vi "Main_PIV_Alex.vi"() -> ()   [LabVIEW 2011]
uses:
  <vilib>/Utility/error.llb/DialogType.ctl
  <vilib>/DAQmx/write.llb/DAQmx Write (Digital Wfm 1Chan NSamp).vi
  <vilib>/DAQmx/write.llb/DAQmx Write (Digital Bool 1Line 1Point).vi
  <vilib>/Waveform/DWDTOps.llb/DWDT Boolean Array to Digital.vi
  <vilib>/DAQmx/create/channels.llb/DAQmx Create Channel (DO-Digital Output).vi
  <vilib>/DAQmx/configure/timing.llb/DAQmx Timing (Sample Clock).vi
  <vilib>/Waveform/DWDTOps.llb/DWDT Uncompress Digital.vi
  <vilib>/DAQmx/miscellaneous.llb/DAQmx Fill In Error Info.vi
  <vilib>/DAQmx/configure/trigger.llb/DAQmx Start Trigger (Digital Edge).vi
panel:
  in  "Tot # of fake flashes 2":i32=50
  out "Pulse Count 2":dbl=50.0
  in  "Loop Time (ms)":u32=100
  in  "Lines 3":tag="Dev1/port0/line0:7" caption="Lines"
  in  "I.C. rate  2":dbl=1000000.0 format="%0.2f"
  out "output array 3":bool[][](array[boolean])
  in  "Pulse 1 Delay 2":u32=500
  in  "On Time 1":u32=1000
  in  "Pulse 2 Delay 2":u32=1500
  in  "On Time 2":u32=1000
  in  "TSI Delay":u32=2
  in  "TSI On Time":u32=10
  out "Image Count":dbl=9.0
  in  "# of I.C. Images":i32=10
  in  "On Tim":u32=300
  in  "Laser 2 delay":u32=1960
  in  "On Time":u32=300
  in  "Laser 1 delay":u32=1910
  out "output array 4":bool[][](array[boolean])
  in  "I.C. Laser rate":dbl=1000000.0 format="%0.2f"
  in  "Lines 4":tag="Dev1/port0/line0:7" caption="Lines"
  in  "TSI":bool=TRUE
  in  "TSI Delay":u32=2
  in  "TSI On Time":u32=10
  in  "Ekspla Laser 2":bool=TRUE
  in  "Laser 2 Delay":u32=1960
  in  "Laser 2 On Time":u32=300
  in  "Ekspla Laser 1":bool=TRUE
  in  "Laser 1 Delay":u32=1910
  in  "Laser 1 On Time":u32=300
  in  "Tot # of fake flashes":i32=49
  out "Pulse Count":dbl=49.0
  in  "Lines 2":tag="Dev1/port0/line0:7" caption="Lines"
  in  "I.C. rate":dbl=1000000.0 format="%0.2f"
  out "output array 2":bool[][](array[boolean])
  in  "Loop Time (ms)":u32=100
  in  "Pulse 1 Delay":u32=500
  in  "On Time":u32=1000
  in  "Pulse 2 Delay":u32=1500
  in  "On Time":u32=1000
  in  "Laser 2 (Fire)":bool
  in  "Laser 1 (Fire)":bool
  in  "FAVs":bool
  in  "Test Trigger":bool
  in  "QS1 On Time":u32
  in  "QS1 Delay":u32
  in  "Fire2 On Time":u32
  in  "Fire2 Delay 3":u32
  in  "QS2 On Time":u32
  in  "QS2 Delay":u32
  in  "Fire1 On Time":u32
  in  "Fire1 Delay 3":u32
  out "output array":bool[][](array[boolean])
  out "Digital Waveform (PCI 6534)":digitalwaveform(graph)={"t0"=timestamp(0 s since 1904-01-01), "dt"=1e-06, "Y"={"transitions"=[], "data"=array3000x8[24000 elements]}}
  in  "Fire Rate":dbl=1000000.0 format="%0.2f"
  in  "Lines":tag="Dev1/port0/line0:7"
  in  "Boolean 24":bool
  in  "End Wall Valve":bool
  in  "Lower Tube E4":bool
  in  "DING":bool
  in  "Lower Tueb E2":bool
  in  "Lowr Tube E1":bool
  in  "Boolean 18":bool
  in  "Boolean 17":bool
  in  "Boolean 16":bool
  in  "Tube LP TV":bool
  in  "Fav #2":bool
  in  "Fav #1":bool
  in  "Vacuum Pump":bool
  in  "Boolean 11":bool
  in  "Diaph Vacuum":bool
  in  "Diaph Supply":bool
  in  "Diaph Vent":bool
  in  "Diaph Master":bool
  in  "Driver LP TV":bool
  in  "Supply Auto V":bool
  in  "Driver Vacuum":bool
  in  "Driver Supply":bool
  in  "Driver Vent":bool
  in  "Driver Master":bool
  in  "stop":bool
  in  "Run Experiment":bool
  # "Shock Tube Controls"
  # "Injectors"
  # "BubbleFill"
  # "Initial Conditions"
  # "Experiment"
  # "SureliteII (need a charge pulse)"
  # "Qswitch/Fire delay: 194us"
  # "Ekspla Charge I.C. (49 fake pulses)"
  # "Fire ---> Qswitch"
  # "i.e. 49"
  # "SureliteII (not needed)"
  # "IC Images"
  # "Ekspla Fire"
  # "TSI"
  # "lase at: 3264 and 3314"
  # "readout time before shock"
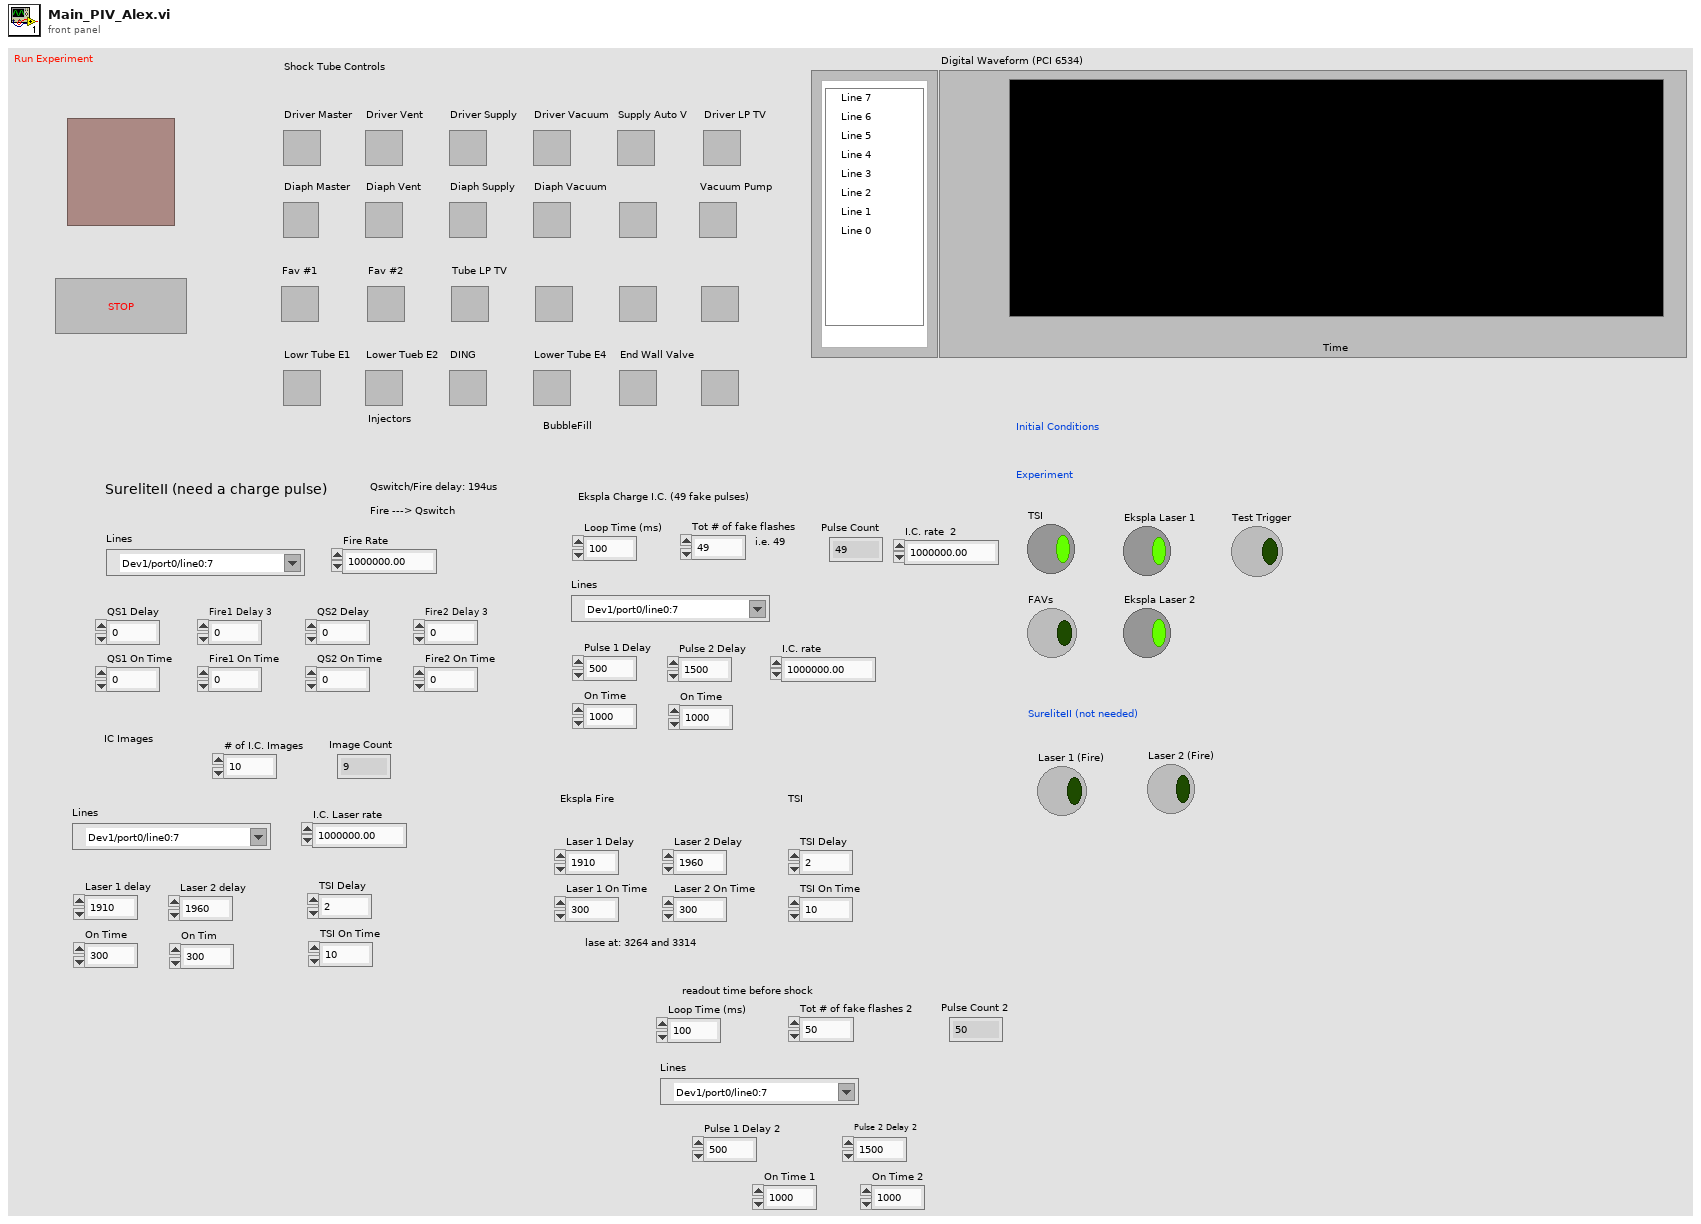
[diagram p1: front panel]
types:
  T1 = typedef "DialogType.ctl" = u16
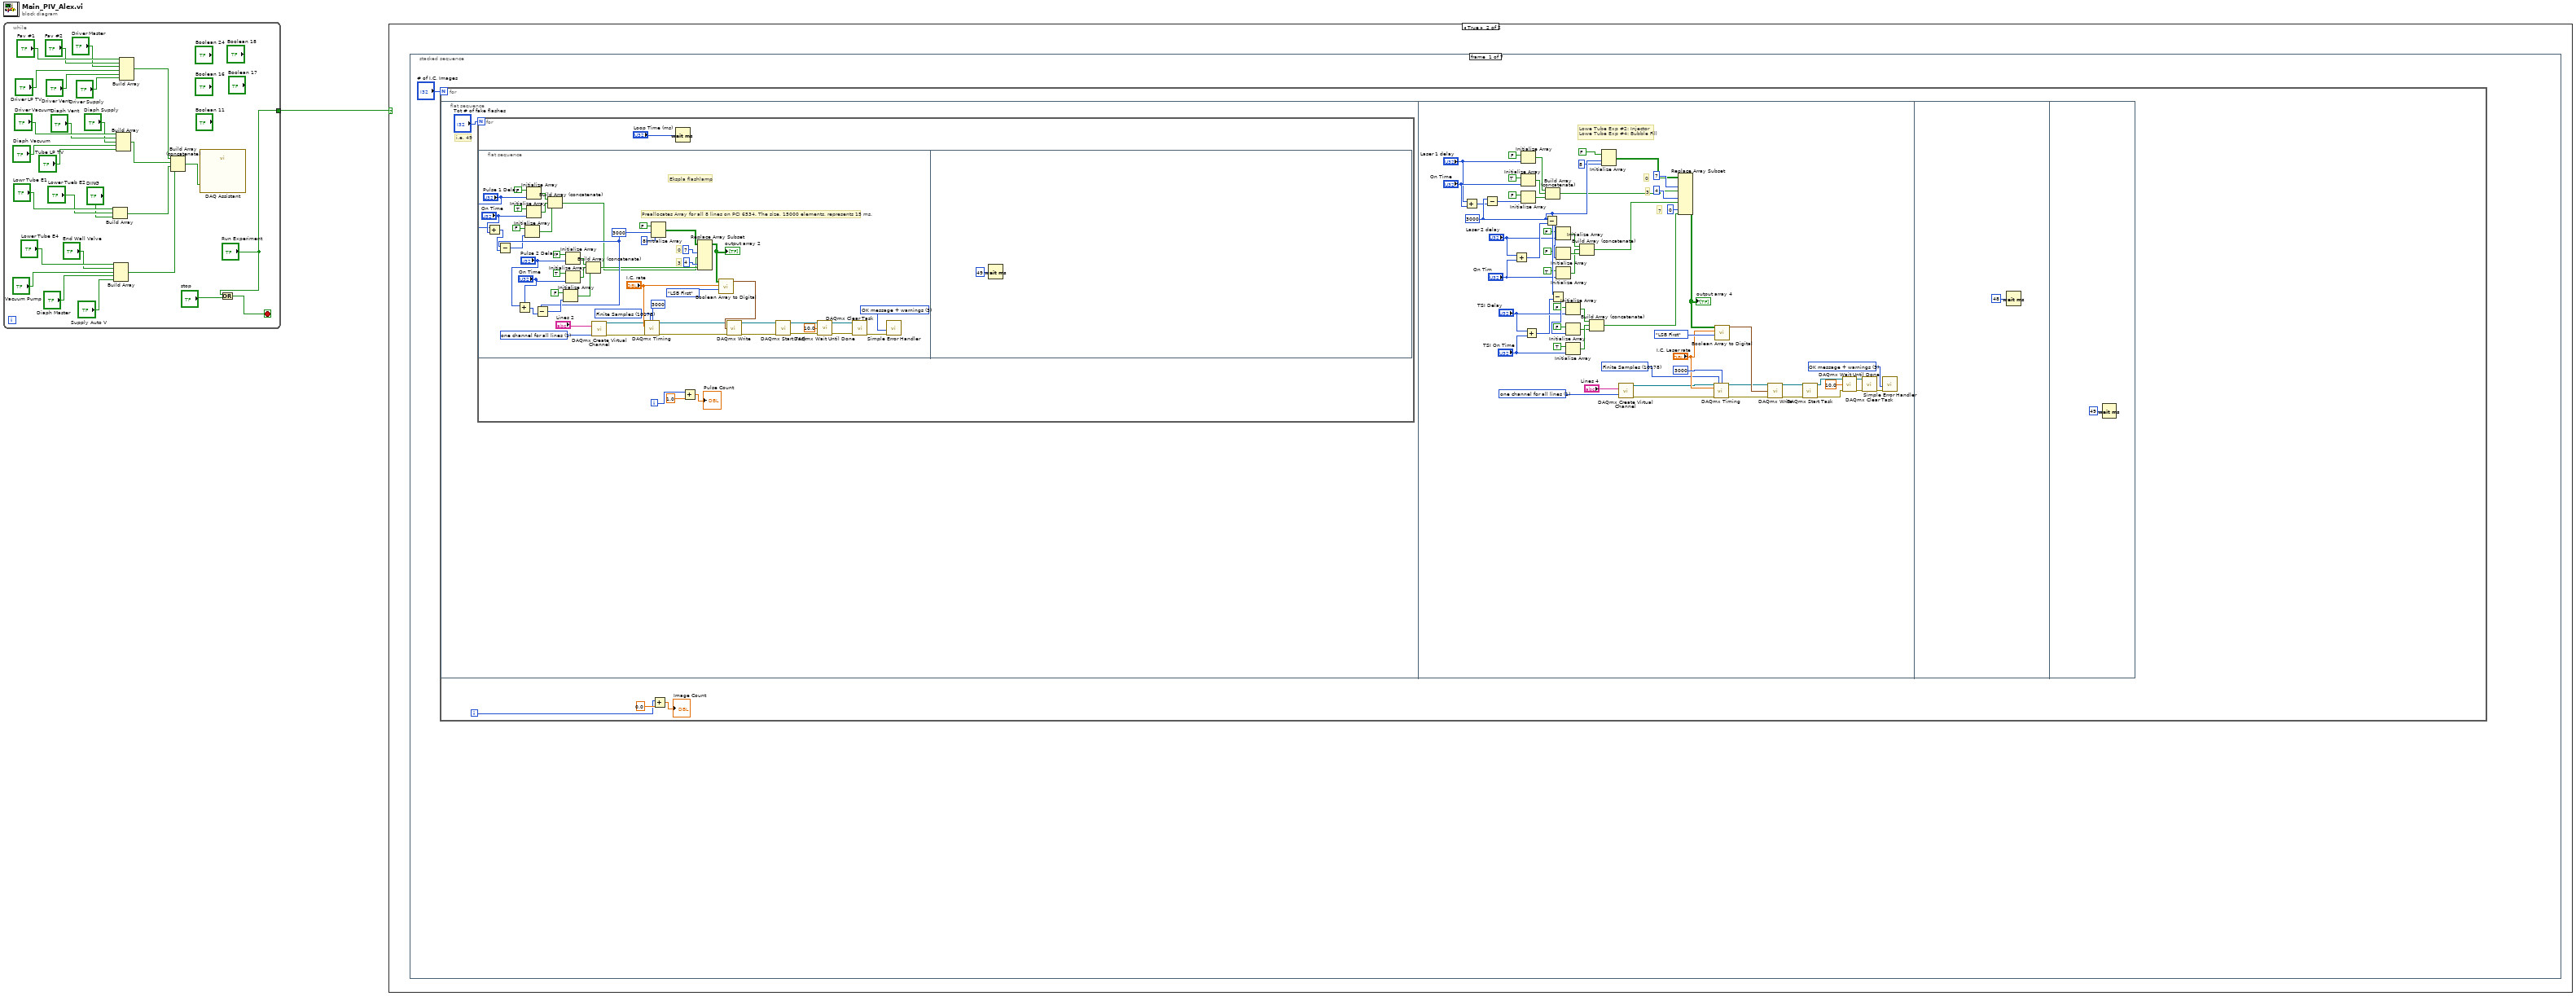
[diagram p0: block diagram]
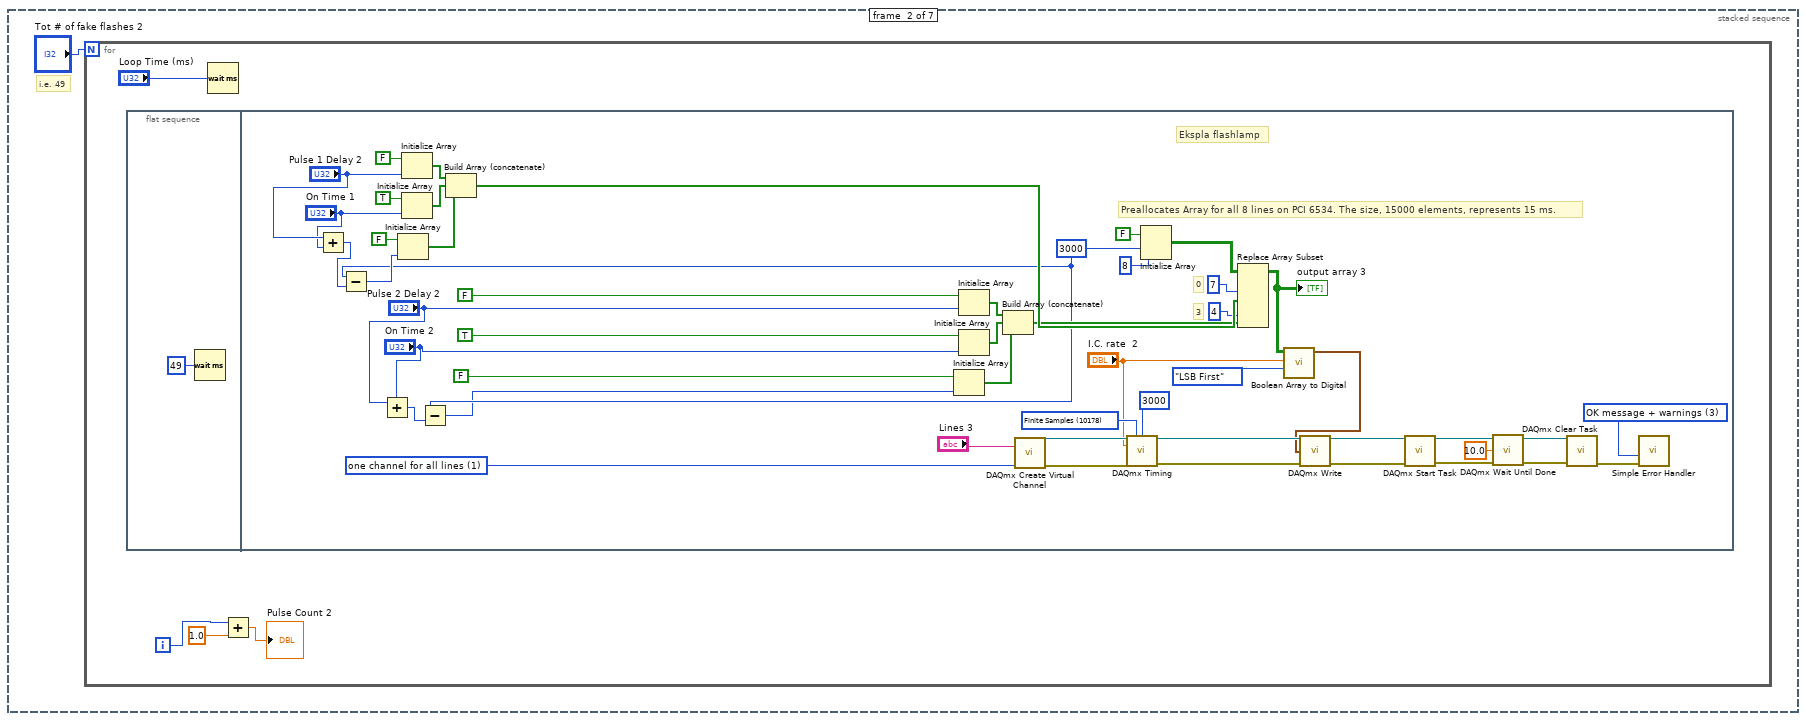
[diagram p3: hidden frame]
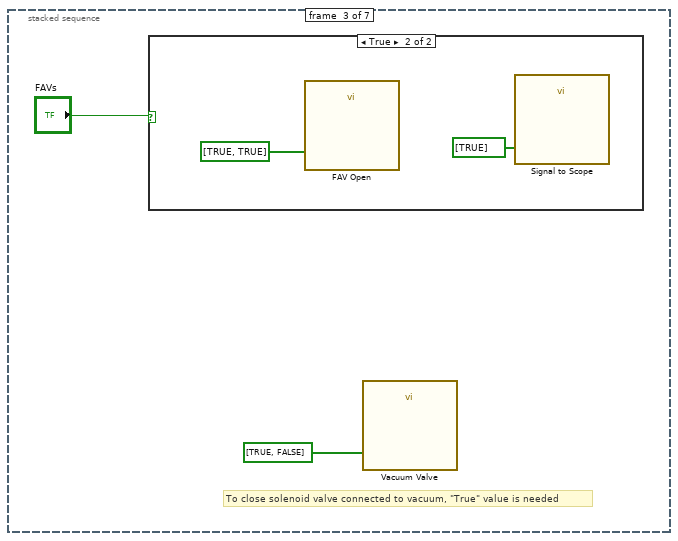
[diagram p4: hidden frame]
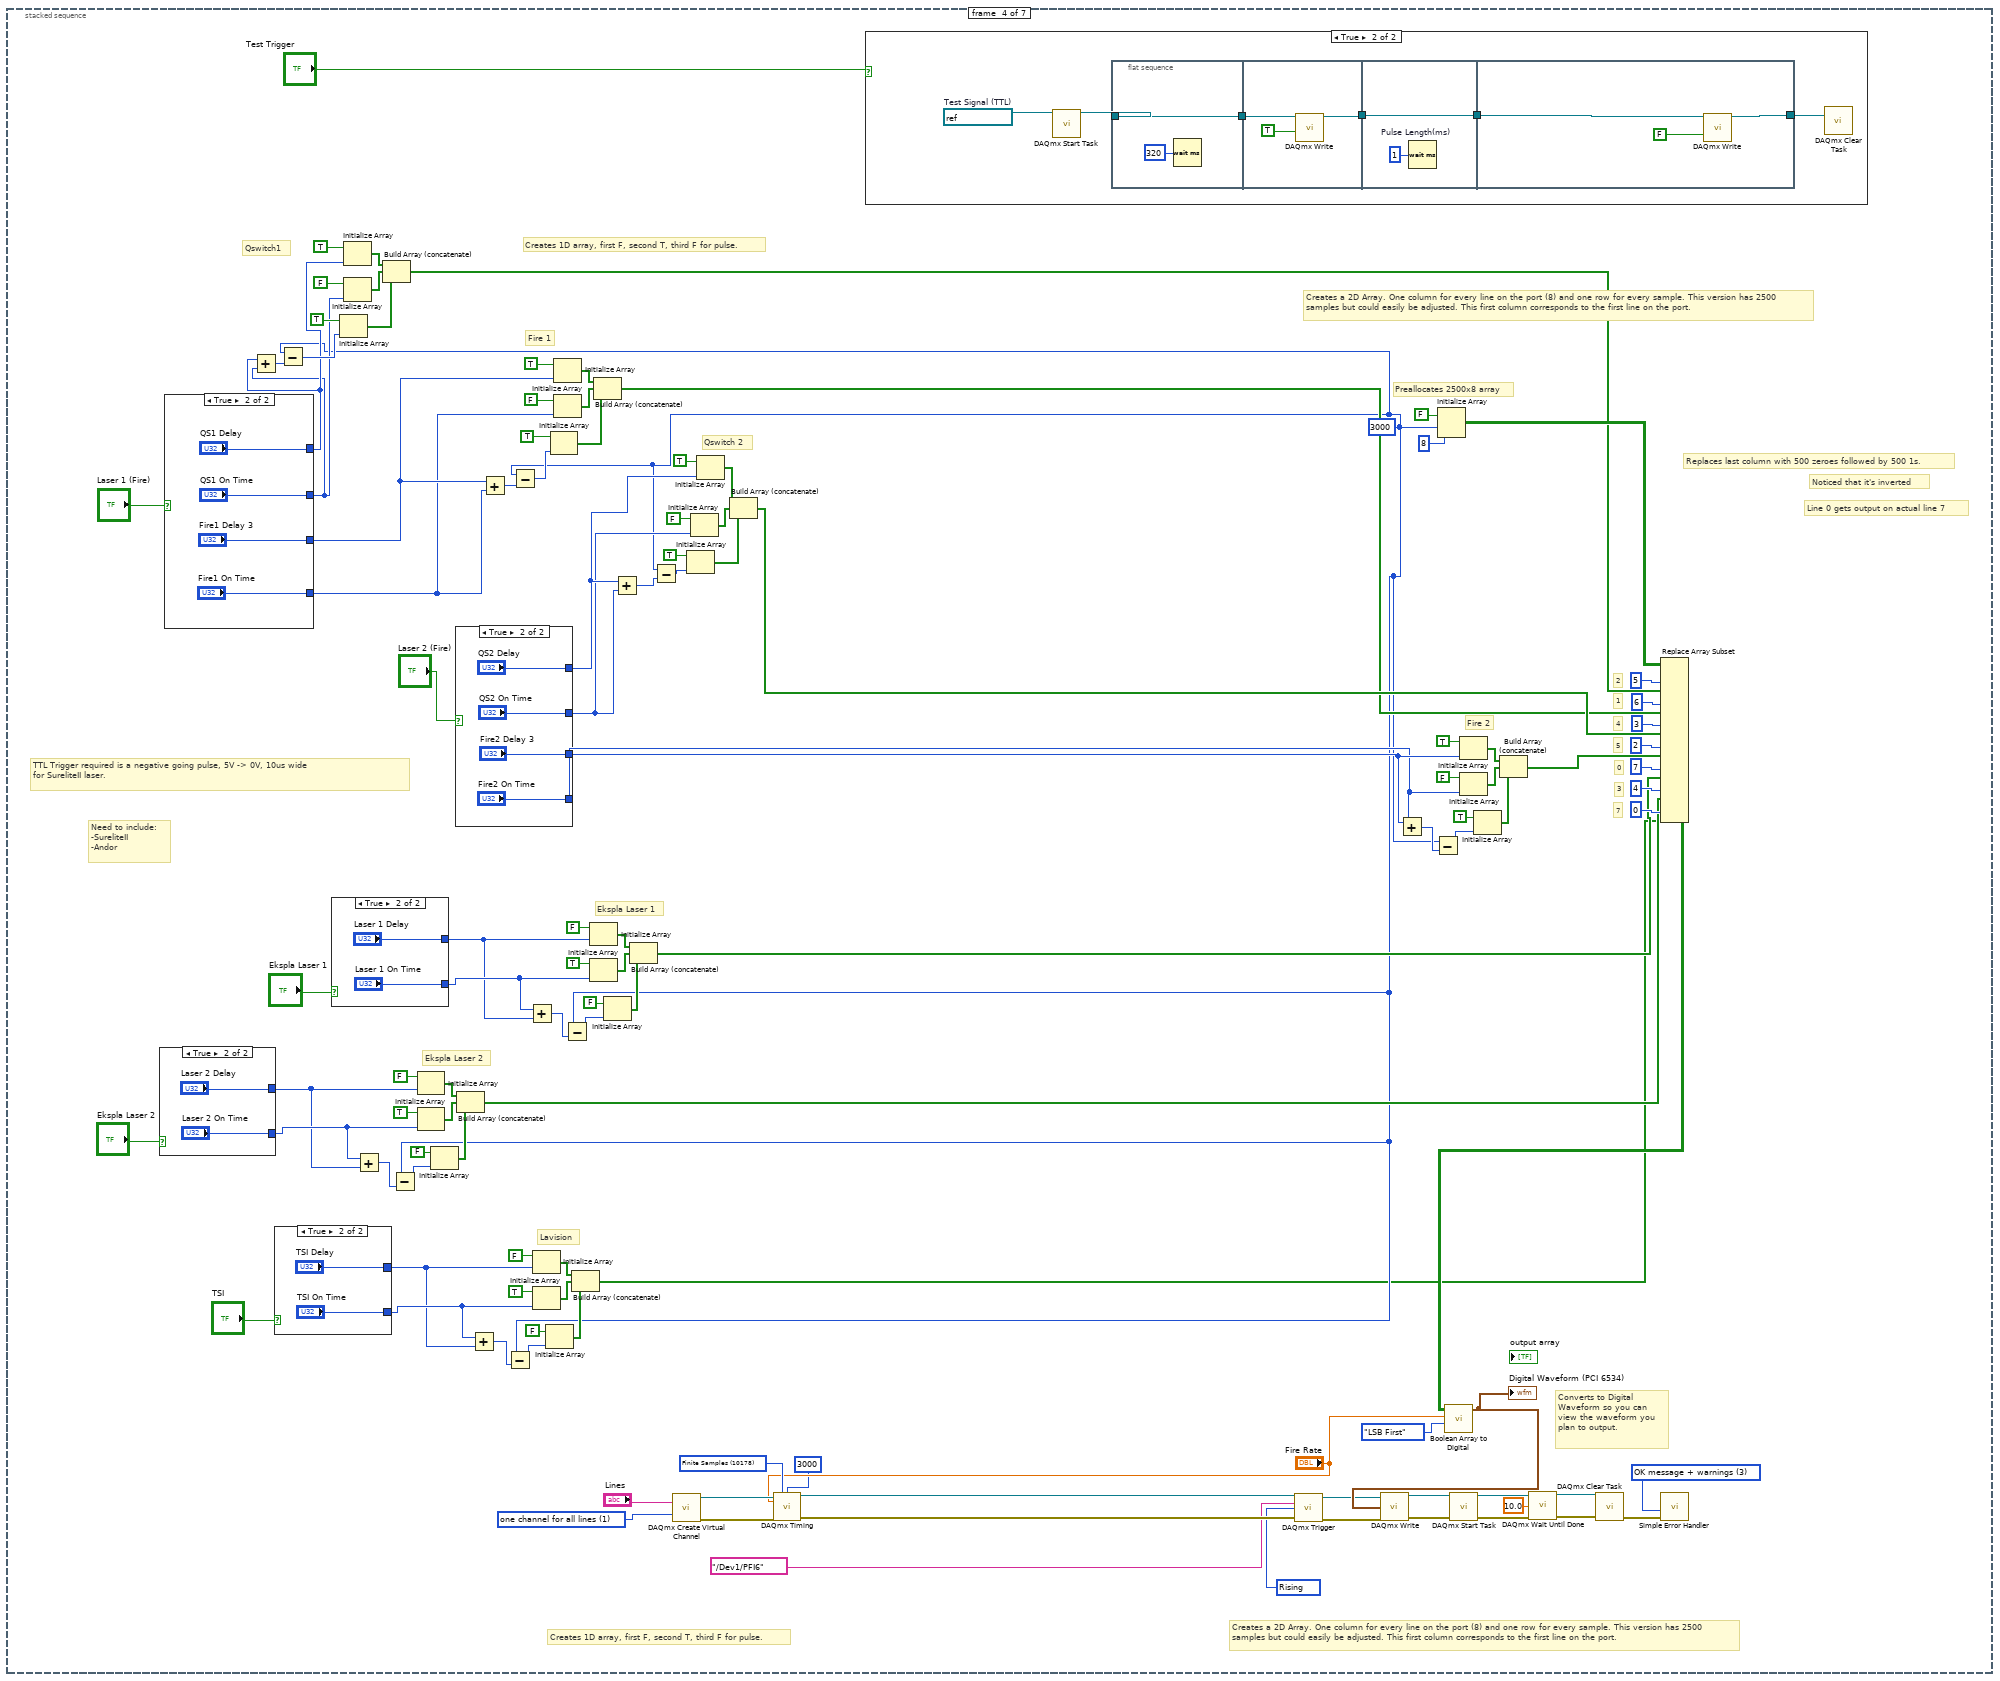
[diagram p6: hidden frame]
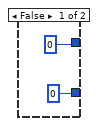
[diagram p7: hidden frame]
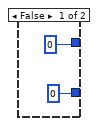
[diagram p8: hidden frame]
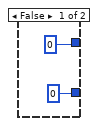
[diagram p9: hidden frame]
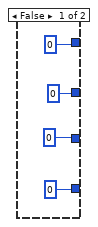
[diagram p10: hidden frame]
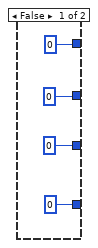
[diagram p11: hidden frame]
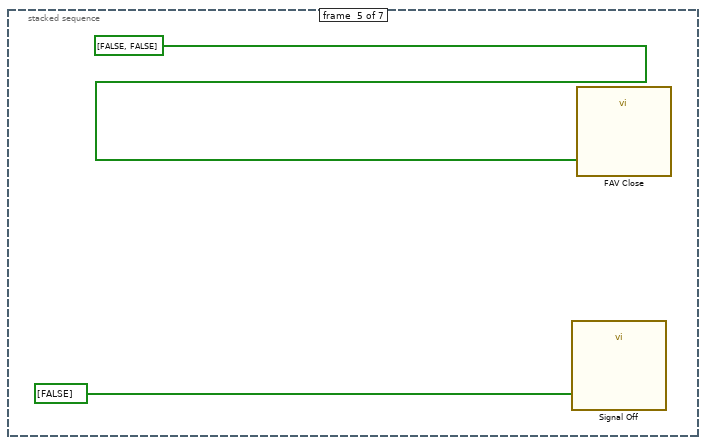
[diagram p13: hidden frame]
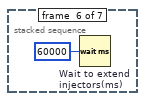
[diagram p14: hidden frame]
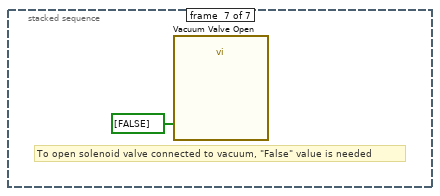
[diagram p15: hidden frame]
diagram:
  n1 = while {
    tunnel: ["Run Experiment"] -> w1
    stop <- w26 stop-if-true
    n2 = Build Array("Lowr Tube E1", "Lower Tueb E2", "DING") -> (w23:bool[])
    n3 = Build Array("Lower Tube E4", "End Wall Valve", "Vacuum Pump", "Diaph Master", "Supply Auto V") -> (w22:bool[])
    n4 = Build Array("Driver Vacuum", "Diaph Vent", "Diaph Supply", "Diaph Vacuum", "Tube LP TV") -> (w24:bool[])
    n5 = Build Array("Fav #1", "Fav #2", "Driver Master", "Driver LP TV", "Driver Vent", "Driver Supply") -> (w25:bool[])
    n6 = Build Array (concatenate)(w25, w24, w23, w22) -> (w2:bool[])
    n7 = call "DAQ Assistant"("data"=w2) -> ()  [unwired: 17 in, 2 out]
    n8 = Or(x="Run Experiment", y="stop") -> (x .or. y?=w26:bool)
  }
  n9 = case shown="True" w1 {
    frame False {
    }
    frame True {
      n10 = stacked-sequence {
        frame #0 {
          n11 = for {
            N: "# of I.C. Images" -> [_]
            i -> [w30]
            n12 = flat-sequence {
              frame #0 {
                # "i.e. 49"
                n13 = for {
                  N: "Tot # of fake flashes" -> [_]
                  i -> [w36]
                  n14 = flat-sequence {
                    frame #0 {
                      w85 = 3000 ("dimension size")
                      w44 = 10178 items=["Finite Samples"=10178, "Continuous Samples"=10123, "Hardware Timed Single Point"=12522] ("sample mode")
                      w41 = 1 items=["one channel for each line", "one channel for all lines"] ("line grouping")
                      w40 = T1 3 items=["no dialog", "OK message", "continue or stop message", "OK message + warnings", "continue/stop + warnings"] ("type of dialog (OK msg:1)")
                      # "0"
                      # "3"
                      # "Ekspla flashlamp"
                      # "Preallocates Array for all 8 lines on PCI 6534. The size, 15000 elements, represents 15 ms."
                      n15 = Add(x="Pulse 1 Delay", y="On Time") -> (x+y=w80:u32)
                      n16 = Subtract(x=w85, y=w80) -> (x-y=w81:u32)
                      n17 = Add(x="Pulse 2 Delay", y="On Time") -> (x+y=w84:u32)
                      n18 = Initialize Array(FALSE, w81) -> (w69:bool[])
                      n19 = Initialize Array(FALSE, "Pulse 1 Delay") -> (w58:bool[])
                      n20 = Initialize Array(TRUE, "On Time") -> (w57:bool[])
                      n21 = Subtract(x=w85, y=w84) -> (x-y=w86:u32)
                      n22 = Build Array (concatenate)(w58, w57, w69) -> (w59:bool[])
                      n23 = Initialize Array(FALSE, w86) -> (w75:bool[])
                      n24 = Initialize Array(FALSE, "Pulse 2 Delay") -> (w73:bool[])
                      n25 = Initialize Array(TRUE, "On Time") -> (w72:bool[])
                      n26 = Build Array (concatenate)(w73, w72, w75) -> (w77:bool[])
                      n27 = call-poly <vilib>:"DAQmx Create Virtual Channel.vi"("lines"="Lines 2", "line grouping"=w41) -> ("task out"=w42:refnum<k21>, "error out"=w43:errorcluster)  [unwired: 12 in]
                      n28 = call-poly <vilib>:"DAQmx Timing.vi"("task/channels in"=w42, "sample mode"=w44, "samples per channel"=3000, "rate"="I.C. rate", "error in"=w43) -> ("task out"=w54:refnum<k21>, "error out"=w55:errorcluster)  [unwired: 9 in]
                      n29 = Initialize Array(FALSE, w85, 8 ("dimension size")) -> (w48:bool[][])
                      n30 = Replace Array Subset(array=w48, new element #1=w59, index (col) #1=7 ("disabled index (col)"), new element #2=w77, index (col) #2=4 ("index (col)")) -> (w51:bool[][])  [unwired: 2 in]
                      "output array 2" <- w51
                      n31 = call-poly <vilib>:"Boolean Array to Digital.vi"("mode"=enum16{"LSB First", "MSB First"}."LSB First", "sample rate"="I.C. rate", "boolean array"=w51) -> ("digital waveform"=w61:digitalwaveform)  [unwired: 7 in, 1 out]
                      n32 = call-poly <vilib>:"DAQmx Write.vi"("task/channels in"=w54, "data"=w61, "error in"=w55) -> ("task out"=w52:refnum<k21>, "error out"=w53:errorcluster)  [unwired: 10 in, 1 out]
                      n33 = call <vilib>:"DAQmx Start Task.vi"("task/channels in"=w52, "error in"=w53) -> ("task out"=w65:refnum<k21>, "error out"=w66:errorcluster)  [unwired: 12 in]
                      n34 = call <vilib>:"DAQmx Wait Until Done.vi"("task/channels in"=w65, "timeout (sec)"=10.0, "error in"=w66) -> ("task out"=w63:refnum<k21>, "error out"=w62:errorcluster)  [unwired: 11 in]
                      n35 = call <vilib>:"DAQmx Clear Task.vi"("task in"=w63, "error in"=w62) -> ("error out"=w38:errorcluster)  [unwired: 13 in]
                      n36 = call <vilib>:"Simple Error Handler.vi"("type of dialog (OK msg:1)"=w40, "error in (no error)"=w38) -> ()  [unwired: 3 in, 5 out]
                    }
                    frame #1 {
                      n37 = Wait (ms)(milliseconds to wait=u32 49) -> ()  [unwired: 1 out]
                    }
                  }
                  n38 = Wait (ms)(milliseconds to wait="Loop Time (ms)") -> ()  [unwired: 1 out]
                  n39 = Add(x=w36, y=1.0) -> (x+y=→"Pulse Count":dbl)
                }
              }
              frame #1 {
                w146 = 3000 ("dimension size")
                w94 = 10178 items=["Finite Samples"=10178, "Continuous Samples"=10123, "Hardware Timed Single Point"=12522] ("sample mode")
                w91 = 1 items=["one channel for each line", "one channel for all lines"] ("line grouping")
                w90 = T1 3 items=["no dialog", "OK message", "continue or stop message", "OK message + warnings", "continue/stop + warnings"] ("type of dialog (OK msg:1)")
                # "7"
                # "0"
                # "3"
                # "Lowe Tube Exp #2: Injector\nLowe Tube Exp #4: Bubble Fill"
                n40 = Add(x="Laser 1 delay", y="On Time") -> (x+y=w130:u32)
                n41 = Subtract(x=w146, y=w130) -> (x-y=w131:u32)
                n42 = Add(x="Laser 2 delay", y="On Tim") -> (x+y=w134:u32)
                n43 = Initialize Array(FALSE, "Laser 1 delay") -> (w108:bool[])
                n44 = Initialize Array(TRUE, "On Time") -> (w107:bool[])
                n45 = Initialize Array(FALSE, w131) -> (w119:bool[])
                n46 = Add(x="TSI Delay", y="TSI On Time") -> (x+y=w135:u32)
                n47 = Subtract(x=w146, y=w134) -> (x-y=w144:u32)
                n48 = Build Array (concatenate)(w108, w107, w119) -> (w109:bool[])
                n49 = Subtract(x=w146, y=w135) -> (x-y=w145:u32)
                n50 = Initialize Array(FALSE, "Laser 2 delay") -> (w123:bool[])
                n51 = Initialize Array(FALSE, w144) -> (w125:bool[])
                n52 = Initialize Array(TRUE, "On Tim") -> (w122:bool[])
                n53 = Initialize Array(FALSE, "TSI Delay") -> (w140:bool[])
                n54 = Initialize Array(FALSE, w145) -> (w138:bool[])
                n55 = Initialize Array(TRUE, "TSI On Time") -> (w141:bool[])
                n56 = Build Array (concatenate)(w123, w122, w125) -> (w127:bool[])
                n57 = Build Array (concatenate)(w140, w141, w138) -> (w147:bool[])
                n58 = Initialize Array(FALSE, w146, 8 ("dimension size")) -> (w98:bool[][])
                n59 = call-poly <vilib>:"DAQmx Create Virtual Channel.vi"("lines"="Lines 4", "line grouping"=w91) -> ("task out"=w92:refnum<k21>, "error out"=w93:errorcluster)  [unwired: 12 in]
                n60 = Replace Array Subset(array=w98, new element #1=w109, index (col) #1=7 ("disabled index (col)"), new element #2=w127, index (col) #2=4 ("index (col)"), new element #3=w147, index (col) #3=0 ("index (col)")) -> (w101:bool[][])  [unwired: 3 in]
                "output array 4" <- w101
                n61 = call-poly <vilib>:"DAQmx Timing.vi"("task/channels in"=w92, "sample mode"=w94, "samples per channel"=3000, "rate"="I.C. Laser rate", "error in"=w93) -> ("task out"=w104:refnum<k21>, "error out"=w105:errorcluster)  [unwired: 9 in]
                n62 = call-poly <vilib>:"Boolean Array to Digital.vi"("mode"=enum16{"LSB First", "MSB First"}."LSB First", "sample rate"="I.C. Laser rate", "boolean array"=w101) -> ("digital waveform"=w111:digitalwaveform)  [unwired: 7 in, 1 out]
                n63 = call-poly <vilib>:"DAQmx Write.vi"("task/channels in"=w104, "data"=w111, "error in"=w105) -> ("task out"=w102:refnum<k21>, "error out"=w103:errorcluster)  [unwired: 10 in, 1 out]
                n64 = call <vilib>:"DAQmx Start Task.vi"("task/channels in"=w102, "error in"=w103) -> ("task out"=w115:refnum<k21>, "error out"=w116:errorcluster)  [unwired: 12 in]
                n65 = call <vilib>:"DAQmx Wait Until Done.vi"("task/channels in"=w115, "timeout (sec)"=10.0, "error in"=w116) -> ("task out"=w113:refnum<k21>, "error out"=w112:errorcluster)  [unwired: 11 in]
                n66 = call <vilib>:"DAQmx Clear Task.vi"("task in"=w113, "error in"=w112) -> ("error out"=w88:errorcluster)  [unwired: 13 in]
                n67 = call <vilib>:"Simple Error Handler.vi"("type of dialog (OK msg:1)"=w90, "error in (no error)"=w88) -> ()  [unwired: 3 in, 5 out]
              }
              frame #2 {
                n68 = Wait (ms)(milliseconds to wait=u32 48) -> ()  [unwired: 1 out]
              }
              frame #3 {
                n69 = Wait (ms)(milliseconds to wait=u32 49) -> ()  [unwired: 1 out]
              }
            }
            n70 = Add(x=w30, y=0.0) -> (x+y=→"Image Count":dbl)
          }
        }
        frame #1 {
          # "i.e. 49"
          n71 = for {
            N: "Tot # of fake flashes 2" -> [_]
            i -> [w154]
            n72 = flat-sequence {
              frame #0 {
                n73 = Wait (ms)(milliseconds to wait=u32 49) -> ()  [unwired: 1 out]
              }
              frame #1 {
                w158 = 3000 ("dimension size")
                w199 = 10178 items=["Finite Samples"=10178, "Continuous Samples"=10123, "Hardware Timed Single Point"=12522] ("sample mode")
                w202 = 1 items=["one channel for each line", "one channel for all lines"] ("line grouping")
                w203 = T1 3 items=["no dialog", "OK message", "continue or stop message", "OK message + warnings", "continue/stop + warnings"] ("type of dialog (OK msg:1)")
                # "0"
                # "3"
                # "Ekspla flashlamp"
                # "Preallocates Array for all 8 lines on PCI 6534. The size, 15000 elements, represents 15 ms."
                n74 = Add(x="Pulse 1 Delay 2", y="On Time 1") -> (x+y=w163:u32)
                n75 = Subtract(x=w158, y=w163) -> (x-y=w162:u32)
                n76 = Add(x="Pulse 2 Delay 2", y="On Time 2") -> (x+y=w159:u32)
                n77 = Initialize Array(FALSE, w162) -> (w174:bool[])
                n78 = Initialize Array(FALSE, "Pulse 1 Delay 2") -> (w185:bool[])
                n79 = Initialize Array(TRUE, "On Time 1") -> (w186:bool[])
                n80 = Subtract(x=w158, y=w159) -> (x-y=w157:u32)
                n81 = Build Array (concatenate)(w185, w186, w174) -> (w184:bool[])
                n82 = Initialize Array(FALSE, w157) -> (w168:bool[])
                n83 = Initialize Array(FALSE, "Pulse 2 Delay 2") -> (w170:bool[])
                n84 = Initialize Array(TRUE, "On Time 2") -> (w171:bool[])
                n85 = Build Array (concatenate)(w170, w171, w168) -> (w166:bool[])
                n86 = call-poly <vilib>:"DAQmx Create Virtual Channel.vi"("lines"="Lines 3", "line grouping"=w202) -> ("task out"=w201:refnum<k21>, "error out"=w200:errorcluster)  [unwired: 12 in]
                n87 = call-poly <vilib>:"DAQmx Timing.vi"("task/channels in"=w201, "sample mode"=w199, "samples per channel"=3000, "rate"="I.C. rate  2", "error in"=w200) -> ("task out"=w189:refnum<k21>, "error out"=w188:errorcluster)  [unwired: 9 in]
                n88 = Initialize Array(FALSE, w158, 8 ("dimension size")) -> (w195:bool[][])
                n89 = Replace Array Subset(array=w195, new element #1=w184, index (col) #1=7 ("disabled index (col)"), new element #2=w166, index (col) #2=4 ("index (col)")) -> (w192:bool[][])  [unwired: 2 in]
                "output array 3" <- w192
                n90 = call-poly <vilib>:"Boolean Array to Digital.vi"("mode"=enum16{"LSB First", "MSB First"}."LSB First", "sample rate"="I.C. rate  2", "boolean array"=w192) -> ("digital waveform"=w182:digitalwaveform)  [unwired: 7 in, 1 out]
                n91 = call-poly <vilib>:"DAQmx Write.vi"("task/channels in"=w189, "data"=w182, "error in"=w188) -> ("task out"=w191:refnum<k21>, "error out"=w190:errorcluster)  [unwired: 10 in, 1 out]
                n92 = call <vilib>:"DAQmx Start Task.vi"("task/channels in"=w191, "error in"=w190) -> ("task out"=w178:refnum<k21>, "error out"=w177:errorcluster)  [unwired: 12 in]
                n93 = call <vilib>:"DAQmx Wait Until Done.vi"("task/channels in"=w178, "timeout (sec)"=10.0, "error in"=w177) -> ("task out"=w180:refnum<k21>, "error out"=w181:errorcluster)  [unwired: 11 in]
                n94 = call <vilib>:"DAQmx Clear Task.vi"("task in"=w180, "error in"=w181) -> ("error out"=w205:errorcluster)  [unwired: 13 in]
                n95 = call <vilib>:"Simple Error Handler.vi"("type of dialog (OK msg:1)"=w203, "error in (no error)"=w205) -> ()  [unwired: 3 in, 5 out]
              }
            }
            n96 = Wait (ms)(milliseconds to wait="Loop Time (ms)") -> ()  [unwired: 1 out]
            n97 = Add(x=w154, y=1.0) -> (x+y=→"Pulse Count 2":dbl)
          }
        }
        frame #2 {
          # "To close solenoid valve connected to vacuum, \"True\" value is needed"
          n98 = case shown="True" "FAVs" {
            frame False {
            }
            frame True {
              n99 = call "FAV Open"("data"=bool[] [TRUE, TRUE]) -> ()  [unwired: 17 in, 2 out]
              n100 = call "Signal to Scope"("data"=bool[] [TRUE]) -> ()  [unwired: 17 in, 2 out]
            }
          }
          n101 = call "Vacuum Valve"("data"=bool[] [TRUE, FALSE]) -> ()  [unwired: 17 in, 2 out]
        }
        frame #3 {
          w281 = 10280 items=["Rising"=10280, "Falling"=10171] ("slope")
          w211 = 3000 ("dimension size")
          w322 = 10178 items=["Finite Samples"=10178, "Continuous Samples"=10123, "Hardware Timed Single Point"=12522] ("sample mode")
          w325 = 1 items=["one channel for each line", "one channel for all lines"] ("line grouping")
          w326 = T1 3 items=["no dialog", "OK message", "continue or stop message", "OK message + warnings", "continue/stop + warnings"] ("type of dialog (OK msg:1)")
          # "Lavision"
          # "Ekspla Laser 2"
          # "Ekspla Laser 1"
          # "7"
          # "3"
          # "0"
          # "Creates 1D array, first F, second T, third F for pulse."
          # "Creates a 2D Array. One column for every line on the port (8) and one row for every sample. This version has 2500 samples but could easily be adjusted. This first column corresponds to the first line on the port."
          # "Need to include:\n-SureliteII\n-Andor"
          # "4"
          # "1"
          # "2"
          # "5"
          # "TTL Trigger required is a negative going pulse, 5V -> 0V, 10us wide\nfor SureliteII laser."
          # "Fire 2"
          # "Qswitch 2"
          # "Fire 1"
          # "Qswitch1"
          # "Line 0 gets output on actual line 7"
          # "Noticed that it's inverted"
          # "Converts to Digital Waveform so you can view the waveform you plan to output."
          # "Creates 1D array, first F, second T, third F for pulse."
          # "Replaces last column with 500 zeroes followed by 500 1s."
          # "Preallocates 2500x8 array"
          # "Creates a 2D Array. One column for every line on the port (8) and one row for every sample. This version has 2500 samples but could easily be adjusted. This first column corresponds to the first line on the port."
          n102 = case shown="True" "Ekspla Laser 2" {
            tunnel: [0 "Laser 2 Delay"] -> w224
            tunnel: [0 "Laser 2 On Time"] -> w225
            frame False {
            }
            frame True {
            }
          }
          n103 = case shown="True" "Laser 1 (Fire)" {
            tunnel: [0 "QS1 Delay"] -> w259
            tunnel: [0 "QS1 On Time"] -> w258
            tunnel: [0 "Fire1 Delay 3"] -> w257
            tunnel: [0 "Fire1 On Time"] -> w256
            frame False {
            }
            frame True {
            }
          }
          n104 = Add(x=w259, y=w258) -> (x+y=w263:u32)
          n105 = case shown="True" "TSI" {
            tunnel: [0 "TSI Delay"] -> w213
            tunnel: [0 "TSI On Time"] -> w214
            frame False {
            }
            frame True {
            }
          }
          n106 = Subtract(x=w211, y=w263) -> (x-y=w262:u32)
          n107 = case shown="True" "Ekspla Laser 1" {
            tunnel: [0 "Laser 1 Delay"] -> w236
            tunnel: [0 "Laser 1 On Time"] -> w237
            frame False {
            }
            frame True {
            }
          }
          n108 = Initialize Array(TRUE, w262) -> (w264:bool[])
          n109 = Initialize Array(TRUE, w259) -> (w266:bool[])
          n110 = Initialize Array(FALSE, w258) -> (w267:bool[])
          n111 = Add(x=w225, y=w224) -> (x+y=w228:u32)
          n112 = Build Array (concatenate)(w266, w267, w264) -> (w261:bool[])
          n113 = Subtract(x=w211, y=w228) -> (x-y=w227:u32)
          n114 = Initialize Array(FALSE, w224) -> (w231:bool[])
          n115 = Initialize Array(TRUE, w225) -> (w232:bool[])
          n116 = Initialize Array(FALSE, w227) -> (w229:bool[])
          n117 = case shown="True" "Laser 2 (Fire)" {
            tunnel: [0 "QS2 Delay"] -> w254
            tunnel: [0 "QS2 On Time"] -> w253
            tunnel: [0 "Fire2 Delay 3"] -> w252
            tunnel: [0 "Fire2 On Time"] -> w251
            frame False {
            }
            frame True {
            }
          }
          n118 = Build Array (concatenate)(w231, w232, w229) -> (w223:bool[])
          n119 = Add(x=w214, y=w213) -> (x+y=w212:u32)
          n120 = Add(x=w257, y=w256) -> (x+y=w286:u32)
          n121 = Subtract(x=w211, y=w212) -> (x-y=w216:u32)
          n122 = Subtract(x=w211, y=w286) -> (x-y=w285:u32)
          n123 = Add(x=w237, y=w236) -> (x+y=w240:u32)
          n124 = Initialize Array(FALSE, w213) -> (w219:bool[])
          n125 = Initialize Array(TRUE, w214) -> (w220:bool[])
          n126 = Initialize Array(FALSE, w216) -> (w217:bool[])
          n127 = Initialize Array(TRUE, w285) -> (w299:bool[])
          n128 = Initialize Array(TRUE, w257) -> (w301:bool[])
          n129 = Initialize Array(FALSE, w256) -> (w302:bool[])
          n130 = Subtract(x=w211, y=w240) -> (x-y=w239:u32)
          n131 = Build Array (concatenate)(w219, w220, w217) -> (w210:bool[])
          n132 = Initialize Array(FALSE, w236) -> (w243:bool[])
          n133 = Initialize Array(TRUE, w237) -> (w244:bool[])
          n134 = Build Array (concatenate)(w301, w302, w299) -> (w282:bool[])
          n135 = Initialize Array(FALSE, w239) -> (w241:bool[])
          n136 = Add(x=w254, y=w253) -> (x+y=w284:u32)
          n137 = Build Array (concatenate)(w243, w244, w241) -> (w235:bool[])
          n138 = Subtract(x=w211, y=w284) -> (x-y=w283:u32)
          n139 = call-poly <vilib>:"DAQmx Create Virtual Channel.vi"("lines"="Lines", "line grouping"=w325) -> ("task out"=w324:refnum<k21>, "error out"=w323:errorcluster)  [unwired: 12 in]
          n140 = Initialize Array(TRUE, w283) -> (w289:bool[])
          n141 = Initialize Array(FALSE, w253) -> (w292:bool[])
          n142 = Initialize Array(TRUE, w254) -> (w291:bool[])
          n143 = Build Array (concatenate)(w291, w292, w289) -> (w287:bool[])
          n144 = call-poly <vilib>:"DAQmx Timing.vi"("task/channels in"=w324, "sample mode"=w322, "samples per channel"=3000, "rate"="Fire Rate", "error in"=w323) -> ("task out"=w298:refnum<k21>, "error out"=w296:errorcluster)  [unwired: 9 in]
          n145 = case shown="True" "Test Trigger" {
            frame False {
            }
            frame True {
              w357 = refnum<k21> "Ch1 9474"  # Test Signal (TTL)
              n146 = call <vilib>:"DAQmx Start Task.vi"("task/channels in"=w357) -> ("task out"=w360:refnum<k21>)  [unwired: 13 in, 1 out]
              n147 = flat-sequence {
                tunnel: w360 -> [w364]
                tunnel: [w364] -> w358
                tunnel: [w366] -> w362
                tunnel: w358 -> [w367]
                tunnel: w362 -> [w369]
                tunnel: [w369] -> w361
                tunnel: [w371] -> w359
                tunnel: w361 -> [w372]
                frame #0 {
                  n148 = Wait (ms)(milliseconds to wait=u32 320) -> ()  [unwired: 1 out]
                }
                frame #1 {
                  n149 = call-poly <vilib>:"DAQmx Write.vi"("task/channels in"=w367, "data"=TRUE) -> ("task out"=w366:refnum<k21>)  [unwired: 11 in, 2 out]
                }
                frame #2 {
                  n150 = Wait (ms) "Pulse Length(ms)"(milliseconds to wait=u32 1) -> ()  [unwired: 1 out]
                }
                frame #3 {
                  n151 = call-poly <vilib>:"DAQmx Write.vi"("task/channels in"=w372, "data"=FALSE) -> ("task out"=w371:refnum<k21>)  [unwired: 11 in, 2 out]
                }
              }
              n152 = call <vilib>:"DAQmx Clear Task.vi"("task in"=w359) -> ()  [unwired: 14 in, 1 out]
            }
          }
          n153 = call-poly <vilib>:"DAQmx Trigger.vi"("task/channels in"=w298, "source"=tag "/Dev1/PFI6", "edge"=w281, "error in"=w296) -> ("task out"=w297:refnum<k21>, "error out"=w295:errorcluster)  [unwired: 10 in]
          n154 = Add(x=w252, y=w251) -> (x+y=w272:u32)
          n155 = Subtract(x=w211, y=w272) -> (x-y=w271:u32)
          n156 = Initialize Array(FALSE, w211, 8 ("dimension size")) -> (w318:bool[][])
          n157 = Initialize Array(TRUE, w252) -> (w275:bool[])
          n158 = Initialize Array(FALSE, w251) -> (w276:bool[])
          n159 = Initialize Array(TRUE, w271) -> (w273:bool[])
          n160 = Build Array (concatenate)(w275, w276, w273) -> (w270:bool[])
          n161 = Replace Array Subset(array=w318, new element #1=w261, index (col) #1=5 ("disabled index (col)"), new element #2=w282, index (col) #2=6 ("index (col)"), new element #3=w287, index (col) #3=3 ("index (col)"), new element #4=w270, index (col) #4=2 ("index (col)"), new element #5=w235, index (col) #5=7 ("index (col)"), new element #6=w223, index (col) #6=4 ("index (col)"), new element #7=w210, index (col) #7=0 ("index (col)")) -> (w316:bool[][])  [unwired: 7 in]
          n162 = call-poly <vilib>:"Boolean Array to Digital.vi"("mode"=enum16{"LSB First", "MSB First"}."LSB First", "sample rate"="Fire Rate", "boolean array"=w316) -> ("digital waveform"=w312:digitalwaveform)  [unwired: 7 in, 1 out]
          "Digital Waveform (PCI 6534)" <- w312
          n163 = call-poly <vilib>:"DAQmx Write.vi"("task/channels in"=w297, "data"=w312, "error in"=w295) -> ("task out"=w315:refnum<k21>, "error out"=w314:errorcluster)  [unwired: 10 in, 1 out]
          n164 = call <vilib>:"DAQmx Start Task.vi"("task/channels in"=w315, "error in"=w314) -> ("task out"=w308:refnum<k21>, "error out"=w307:errorcluster)  [unwired: 12 in]
          n165 = call <vilib>:"DAQmx Wait Until Done.vi"("task/channels in"=w308, "timeout (sec)"=10.0, "error in"=w307) -> ("task out"=w310:refnum<k21>, "error out"=w311:errorcluster)  [unwired: 11 in]
          n166 = call <vilib>:"DAQmx Clear Task.vi"("task in"=w310, "error in"=w311) -> ("error out"=w328:errorcluster)  [unwired: 13 in]
          n167 = call <vilib>:"Simple Error Handler.vi"("type of dialog (OK msg:1)"=w326, "error in (no error)"=w328) -> ()  [unwired: 3 in, 5 out]
        }
        frame #4 {
          n168 = call "Signal Off"("data"=bool[] [FALSE]) -> ()  [unwired: 17 in, 2 out]
          n169 = call "FAV Close"("data"=bool[] [FALSE, FALSE]) -> ()  [unwired: 17 in, 2 out]
        }
        frame #5 {
          n170 = Wait (ms) "Wait to extend injectors(ms)"(milliseconds to wait=u32 60000) -> ()  [unwired: 1 out]
        }
        frame #6 {
          # "To open solenoid valve connected to vacuum, \"False\" value is needed"
          n171 = call "Vacuum Valve Open"("data"=bool[] [FALSE]) -> ()  [unwired: 17 in, 2 out]
        }
      }
    }
  }
